vi "TSM SSC Digital Configure HRAM.vi"(0 "Digital TSM In":T1, 7 "HRAM Configuration":T3={"Finite Samples"=TRUE, "Cycles to Acquire"=2303, "Max Samples To Acquire Per Site"=8191, "Buffer Size Per Site"=32000, "Pretrigger Samples"=0, "Trigger Settings"={"Trigger Type"=2200, "Cycle Number Trigger:Cycle Number"=0, "Pattern Label Trigger:Pattern Label"="", "Pattern Label Trigger:Vector Offset"=0, "Pattern Label Trigger:Cycle Offset"=0}} {"Trigger Settings"."Trigger Type" items=["First Failure"=2200, "Cycle Number"=2201, "Pattern Label"=2202]; "Cycles to Acquire" items=["Failed Cycles"=2303, "All Cycles"=2304]}, 11 "error in":errorcluster) -> (4 "Digital TSM Out":T1, 15 "error out":errorcluster)   [LabVIEW 2020]
uses:
  TSM/TSM SSC Digital.ctl
  <vilib>/NI_TestStand_SemiconductorModule/NI_TestStand_Semiconductor_Module.lvlibp/PinMap/Digital Pattern/PinQueryContext/DigitalPatternPinQueryContext.lvclass
  SSC Digital/SSC Digital.ctl
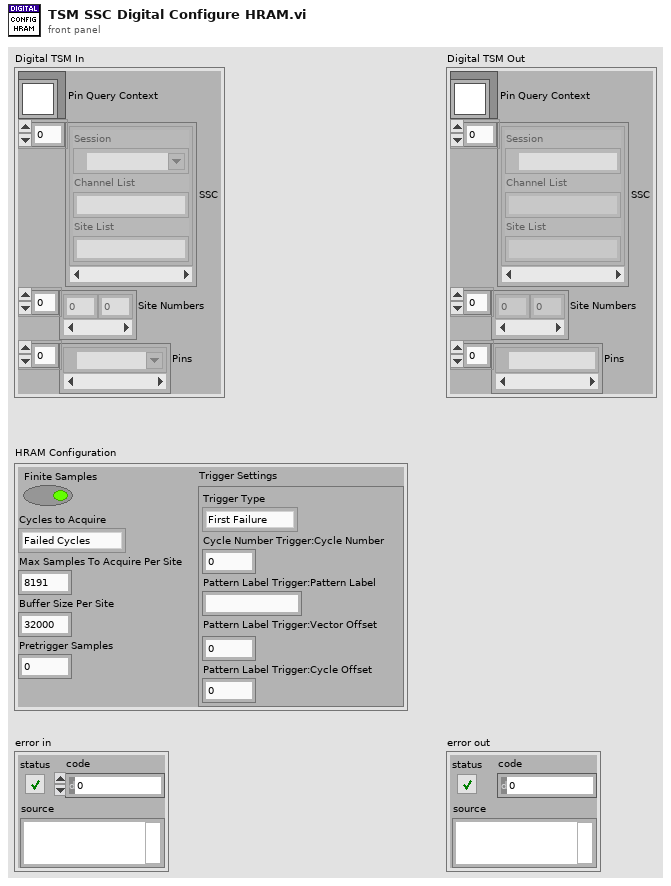
[diagram p1: front panel]
types:
  T1 = typedef "TSM SSC Digital.ctl" = cluster{"Pin Query Context":refnum<class "DigitalPatternPinQueryContext.lvclass">, "SSC":T2[], "Site Numbers":i32[], "Pins":tag[]}
  T2 = typedef "SSC Digital.ctl" = cluster{"Session":refnum<k15>, "Channel List":string, "Site List":string}
  T3 = cluster{"Finite Samples":bool, "Cycles to Acquire":i32, "Max Samples To Acquire Per Site":i32, "Buffer Size Per Site":i64, "Pretrigger Samples":i32, "Trigger Settings":cluster{"Trigger Type":i32, "Cycle Number Trigger:Cycle Number":i64, "Pattern Label Trigger:Pattern Label":string, "Pattern Label Trigger:Vector Offset":i64, "Pattern Label Trigger:Cycle Offset":i64}}
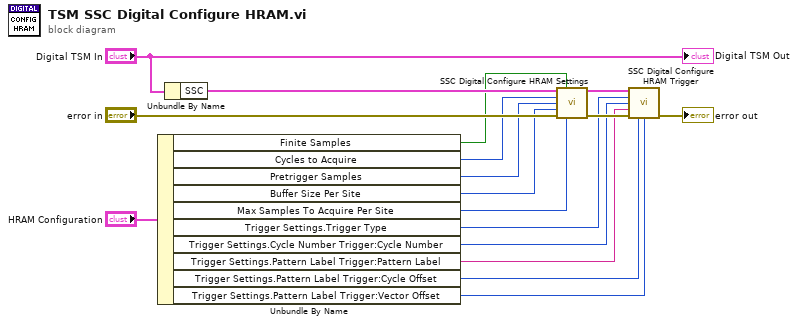
[diagram p0: block diagram]
diagram:
  n1 = Unbundle By Name("HRAM Configuration") -> ("Finite Samples"=w14:bool, "Cycles to Acquire"=w13:i32, "Pretrigger Samples"=w12:i32, "Buffer Size Per Site"=w11:i64, "Max Samples To Acquire Per Site"=w10:i32, "Trigger Settings.Trigger Type"=w5:i32, "Trigger Settings.Cycle Number Trigger:Cycle Number"=w4:i64, "Trigger Settings.Pattern Label Trigger:Pattern Label"=w3:string, "Trigger Settings.Pattern Label Trigger:Cycle Offset"=w2:i64, "Trigger Settings.Pattern Label Trigger:Vector Offset"=w1:i64)
  n2 = Unbundle By Name("Digital TSM In") -> ("SSC"=w16:T2[])
  n3 = call "SSC Digital Configure HRAM Settings.vi"("Digital SSC in"=w16, "Number of Samples is Finite"=w14, "Cycles to Acquire"=w13, "Pretrigger Samples"=w12, "Buffer Size Per Site"=w11, "error in"="error in", "Max Samples To Acquire Per Site"=w10) -> ("Digital SSC out"=w6:T2[], "error out"=w8:errorcluster)  [unwired: 7 in]
  n4 = call "SSC Digital Configure HRAM Trigger.vi"("Digital SSC in"=w6, "Triggers Type"=w5, "Cycle Number Trig:Cycle Number"=w4, "Pattern Label Trig:Pattern Label"=w3, "error in"=w8, "Pattern Label Trig:Cycle Offset"=w2, "Pattern Label Trig:Vector Offset"=w1) -> ("error out"=→"error out":errorcluster)  [unwired: 7 in, 1 out]
  "Digital TSM Out" <- "Digital TSM In"
